vi "Initialize DMA.vi"(7 "Number of Channels":u8, 8 "error in (no error)":errorcluster, 9 "dt":dbl, 10 "Refs":T1={"Data Type"=enum."I32", "DMA_SGL"=refnum, "DMA_U64"=refnum, "DMA_I64"=refnum, "DMA_FXP+/-32.8"=refnum, "DMA_FXP+/-64.32"=refnum, "DMA_U32"=refnum, "DMA_U16"=refnum, "DMA_U8"=refnum, "DMA_I32"=refnum, "DMA_I16"=refnum, "DMA_I8"=refnum, "DMA_FXP+/-32.16"=refnum} {"Data Type" format="%.0x"}, 11 "Multiple Waveforms Write (DBL) in":refnum<class "Multiple Waveforms Write (DBL).lvclass">) -> (0 "error out":errorcluster, 2 "Refs":T1={"Data Type"=enum."I32", "DMA_SGL"=refnum, "DMA_U64"=refnum, "DMA_I64"=refnum, "DMA_FXP+/-32.8"=refnum, "DMA_FXP+/-64.32"=refnum, "DMA_U32"=refnum, "DMA_U16"=refnum, "DMA_U8"=refnum, "DMA_I32"=refnum, "DMA_I16"=refnum, "DMA_I8"=refnum, "DMA_FXP+/-32.16"=refnum} {"Data Type" format="%.0x"}, 3 "Multiple Waveforms Write (DBL) out":refnum<class "Multiple Waveforms Write (DBL).lvclass">)   [LabVIEW 2019, in "FPGA Addon Engine.lvlib"]
uses:
  FPGA Addon Engine.lvlib
  Types/DMA Input Refs.ctl
  Addon Shared/Data Type.ctl
  <vilib>/NI VeriStand/Custom Device Waveform API/Multiple Waveforms Write (DBL)/Multiple Waveforms Write (DBL).lvclass
  C:/Program Files (x86)/National Instruments/LabVIEW 2019/vi.lib/NI VeriStand/Custom Device Waveform API/Waveform Session.lvclass
  <vilib>/NI VeriStand/Custom Device Waveform API/Waveform Session.lvclass/Waveform Session.ctl
  <vilib>/NI VeriStand/Custom Device Waveform API/Multiple Waveforms Write (DBL)/Multiple Waveforms Write (DBL).lvclass/Multiple Waveforms Write (DBL).ctl
  <vilib>/NI VeriStand/Custom Device Waveform API/Internal Comm Classes/WPL Comm/WPL Comm.lvclass/WPL Comm.ctl
  <vilib>/NI VeriStand/Custom Device Waveform API/Multiple Waveforms Write (DBL)/NI VeriStand - Start Multiple Waveforms (DBL).vi
  <vilib>/NI VeriStand/Custom Device Waveform API/Internal Comm Classes/WPL Comm/WPL_start dbl waveform.vi
  <vilib>/NI VeriStand/Custom Device Waveform API/Read Sample offset DVR.vi
  <vilib>/NI VeriStand/Custom Device Waveform API/Check Opened.vi
  <vilib>/NI VeriStand/Custom Device Waveform API/Internal Comm Classes/WPL Comm/Set t0 on Variant.vi
  <vilib>/NI VeriStand/Custom Device Waveform API/Internal Comm Classes/WPL Comm/Send WPL Command.vi
  <vilib>/NI VeriStand/Custom Device Waveform API/Internal Comm Classes/WPL Comm/Convert Q Error to Shutdown Error.vi
  <vilib>/NI VeriStand/Custom Device Waveform API/Internal Comm Classes/WPL Comm/WPL Comm (2D DBL)/WPL Comm (2D DBL).lvclass
  C:/Program Files (x86)/National Instruments/LabVIEW 2019/vi.lib/NI VeriStand/Custom Device Waveform API/Internal Comm Classes/WPL Comm/WPL Comm.lvclass
  <vilib>/Utility/error.llb/Error Cluster From Error Code.vi
  <vilib>/NI VeriStand/Custom Device Waveform API/NI_VS Custom Device Waveform API.lvlib
  Addon Shared/FPGA Addon Shared.lvlib
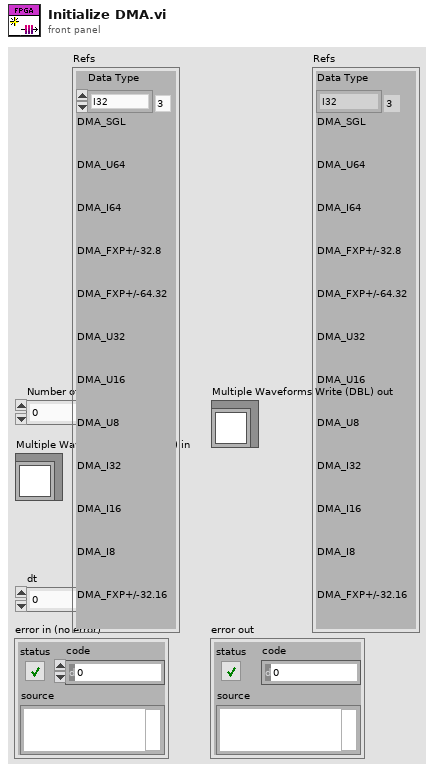
[diagram p1: front panel]
types:
  T1 = typedef "FPGA Addon Engine.lvlib/DMA Input Refs.ctl" = cluster{"Data Type":T2, "DMA_SGL":refnum<k20>, "DMA_U64":refnum<k20>, "DMA_I64":refnum<k20>, "DMA_FXP+/-32.8":refnum<k20>, "DMA_FXP+/-64.32":refnum<k20>, "DMA_U32":refnum<k20>, "DMA_U16":refnum<k20>, "DMA_U8":refnum<k20>, "DMA_I32":refnum<k20>, "DMA_I16":refnum<k20>, "DMA_I8":refnum<k20>, "DMA_FXP+/-32.16":refnum<k20>}
  T2 = typedef "FPGA Addon Shared.lvlib/Data Type.ctl" = enum8{"<Null>", "I8", "I16", "I32", "I64", "U8", "U16", "U32", "U64", "SGL", "Boolean", "Analog PWM In Settings", "Analog PWM In", "Digital PWM In Settings", "Digital PWM In", "Digital PWM Out", "Sine Out", "FXP+/-24.5", "FXP+/-16.5", "FXP+/-32.8", "FXP+/-64.32", "FXP+/-16.7", "FXP+/-20.5", "FXP+/-27.5", "FXP+/-32.16", "FXP +16.3", "FXP +18.3", "Digital Static In", "Digital Static Out", "Digital Static In Settings", "Digital WSS Out", "Quad Encoder Settings", "Quad Encoder In"}
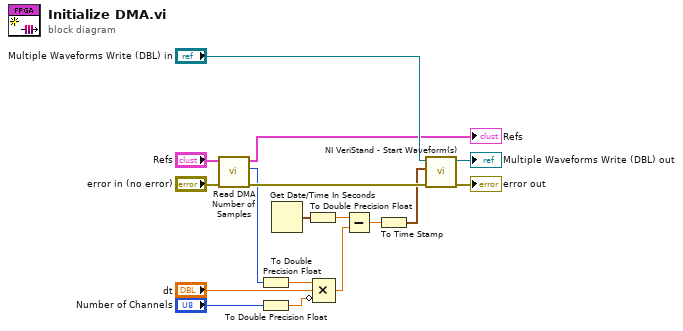
[diagram p0: block diagram]
diagram:
  n1 = call "Read DMA Number of Samples.vi"("error in (no error)"="error in (no error)", "Refs in"="Refs") -> ("error out"=w13:errorcluster, "Elements Remaining"=w7:u32, "Refs out"=→"Refs":T1)  [unwired: 7 in]
  n2 = To Double Precision Float(number=w7) -> (double precision float=w8:dbl)
  n3 = To Double Precision Float(number="Number of Channels") -> (double precision float=w6:dbl)
  n4 = Get Date/Time In Seconds() -> (seconds since 1Jan1904=w5:timestamp)
  n5 = To Double Precision Float(number=w5) -> (double precision float=w3:dbl)
  n6 = Compound Arithmetic op=MULTIPLY(w8, "dt", invert w6) -> (w4:dbl)
  n7 = Subtract(x=w3, y=w4) -> (x-y=w9:dbl)
  n8 = To Time Stamp(1:w9) -> (0:w12:timestamp)
  n9 = call-poly <vilib>:"NI VeriStand - Start Waveform(s).vi"("error in (no error)"=w13, "t0"=w12, "Multiple Waveforms Write Session (DBL) in"="Multiple Waveforms Write (DBL) in") -> ("error out"=→"error out":errorcluster, "Multiple Waveforms Write Session (DBL) out"=→"Multiple Waveforms Write (DBL) out":refnum<class "Multiple Waveforms Write (DBL).lvclass">)  [unwired: 7 in]
